vi "WebAppFGV.vi"() -> ()   [LabVIEW 2019]
uses:
  WebAppDataAction.ctl
panel:
  in  "WebAppFGVAction":T1
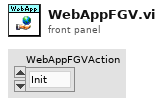
[diagram p1: front panel]
types:
  T1 = typedef "WebAppDataAction.ctl" = enum16{"Init", "Read", "Write", "Release"}
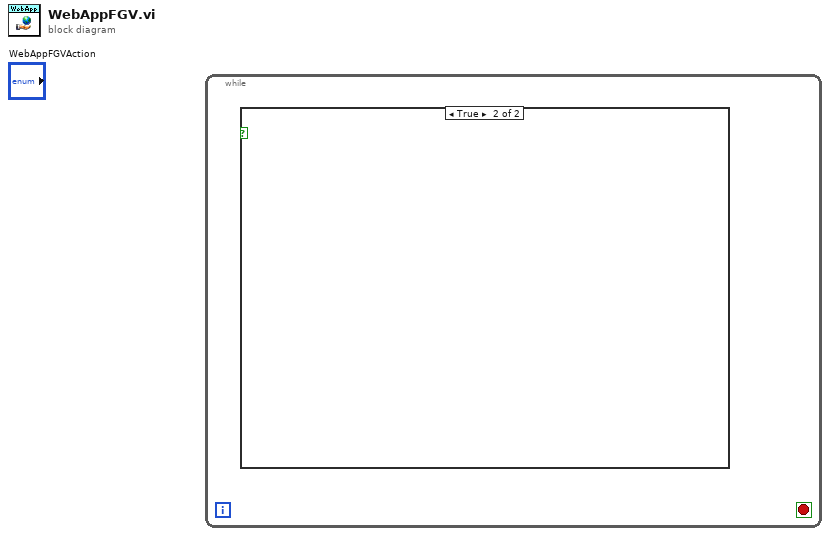
[diagram p0: block diagram]
diagram:
  n1 = while {
    stop <- _ stop-if-true
    n2 = case shown="True" {
      selector: _ -> [_ _]
      frame False {
      }
      frame True {
      }
    }
  }
